vi "Iterate.vi"(8 "error in (no error)":errorcluster, 10 "Iterator Settings":T1={"Prepare timeout (ms)"=200, "Iterate timeout (ms)"=50, "Conclude timeout (ms)"=200, "Iterate period (ms)"=200, "Number of iterations"=5, "Time before stop (ms)"=5, "Active Stop Conditions"={"Number of Iterations"=FALSE, "Time Elapsed"=FALSE, "Iteration Result"=FALSE}, "Prepare Msg"=refnum, "Iterate Msg"=refnum, "Conclude Msg"=refnum, "Iterations End Report"=refnum}, 11 "Iterator Actor in":refnum<class "Iterator NR Actor.lvclass">) -> (0 "error out":errorcluster, 3 "Iterator Actor out":refnum<class "Iterator NR Actor.lvclass">)   [LabVIEW 2023, in "Iterator Actor.lvlib" / "Iterator NR Actor.lvclass"]
doc: "Iteratively calls the Iterate method of the Client. \nStops the iterations either by receiving the Stop signal, or by any of predefined Stop conditions."
uses:
  Iterator NR Actor.lvclass
  Abstract Iterator Actor/Iterator Settings.ctl
  Iterator Actor/Iterator Actor Abstract Messages/Iterator Report Iterations End Msg/Iterator Report Iterations End Msg.lvclass
  <vilib>/ActorFramework/Message/Message.lvclass
  Abstract Iterator Actor/Active Stop Conditions.ctl
  Abstract Iterator Actor/Abstract Iterator Actor.lvclass/Abstract Iterator Actor.ctl
  Abstract Iterator Actor/Stop Reason.ctl
  <vilib>/ActorFramework/Actor/Actor.lvclass/Actor.ctl
  <vilib>/ActorFramework/Message Enqueuer/Message Enqueuer.lvclass/Message Enqueuer.ctl
  Iterator NR Actor.lvclass/Iterator NR Actor.ctl
  <vilib>/ActorFramework/Batch Msg/Batch Msg.lvclass/Batch Msg.ctl
  Abstract Iterator Actor/Iterator Errors.ctl
  Abstract Iterator Actor/Read Stop Iterate Notifier.vi
  <vilib>/ActorFramework/Message Enqueuer/Init from Existing Queue.vi
  <vilib>/ActorFramework/Actor/Read Caller Enqueuer.vi
  <vilib>/ActorFramework/Batch Msg/Send Batch.vi
  <vilib>/ActorFramework/Message Enqueuer/Enqueue.vi
  Iterator NR Actor Messages/Request Iteration Notification Msg/Request Iteration Notification Msg.lvclass
  <vilib>/ActorFramework/Batch Msg/Batch Msg.lvclass
  <userlib>/_OpenG.lib/lvdata/lvdata.llb/LVOOP Is Same Or Descendant Class__ogtk.vi
  <vilib>/ActorFramework/Message Priority Queue/Priority Enqueue.vi
  <vilib>/ActorFramework/Message Enqueuer/Message Enqueuer.lvclass
  Iterator NR Actor Messages/Iteration Msg/Abstract Iteration Msg.lvclass
  <userlib>/_OpenG.lib/time/time.llb/openg_time.lvlib
  Iterator Actor/Iterator Actor Messages/Write Stop Reason Msg/Write Stop Reason Msg.lvclass
  <vilib>/ActorFramework/Actor/Actor.lvclass
  Abstract Iterator Actor/Abstract Iterator Actor.lvclass
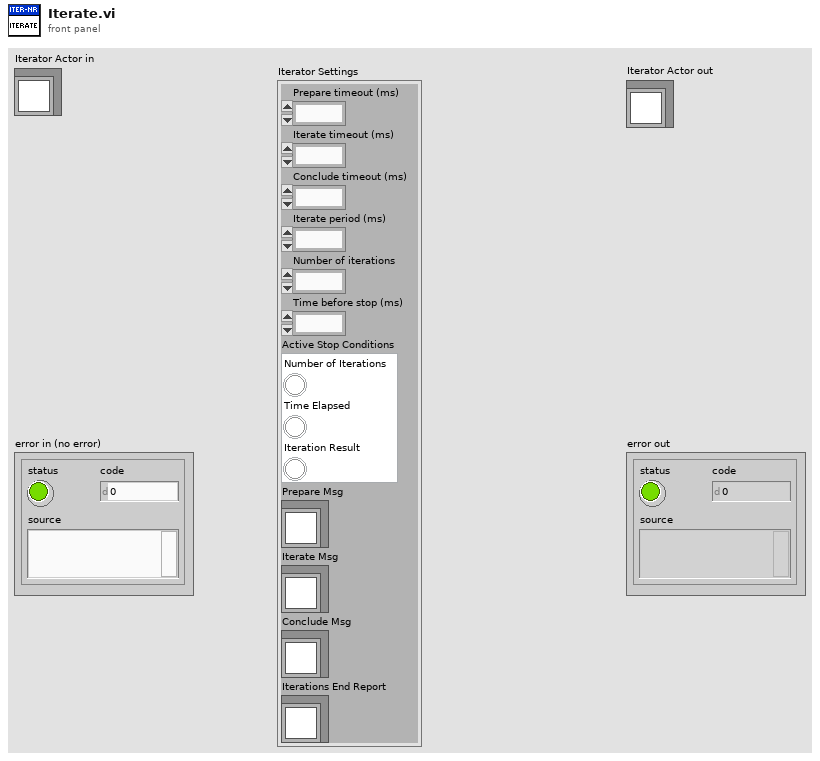
[diagram p1: front panel]
types:
  T1 = typedef "Iterator Actor.lvlib/Abstract Iterator Actor.lvclass/Iterator Settings.ctl" = cluster{"Prepare timeout (ms)":i32, "Iterate timeout (ms)":i32, "Conclude timeout (ms)":i32, "Iterate period (ms)":i32, "Number of iterations":i32, "Time before stop (ms)":i32, "Active Stop Conditions":T2, "Prepare Msg":refnum<class "Message.lvclass">, "Iterate Msg":refnum<class "Message.lvclass">, "Conclude Msg":refnum<class "Message.lvclass">, "Iterations End Report":refnum<class "Iterator Report Iterations End Msg.lvclass">}
  T2 = typedef "Iterator Actor.lvlib/Abstract Iterator Actor.lvclass/Active Stop Conditions.ctl" = cluster{"Number of Iterations":bool, "Time Elapsed":bool, "Iteration Result":bool}
  T3 = typedef "Iterator Actor.lvlib/Abstract Iterator Actor.lvclass/Stop Reason.ctl" = enum16{"Number of Iterations", "Time Elapsed", "Stopped Internally", "Stopped Externally"}
  T4 = typedef "Iterator Actor.lvlib/Abstract Iterator Actor.lvclass/Iterator Errors.ctl" = enum16{"Input parameters are not valid", "Preparation call timed out", "Iteration call timed out", "Conclusion call timed out"}
  T5 = typedef "Iterator Actor.lvlib/Abstract Iterator Actor.lvclass/Stop Condition.ctl" = enum16{"None", "Number of Iterations", "Time Elapsed", "Iteration Result"}
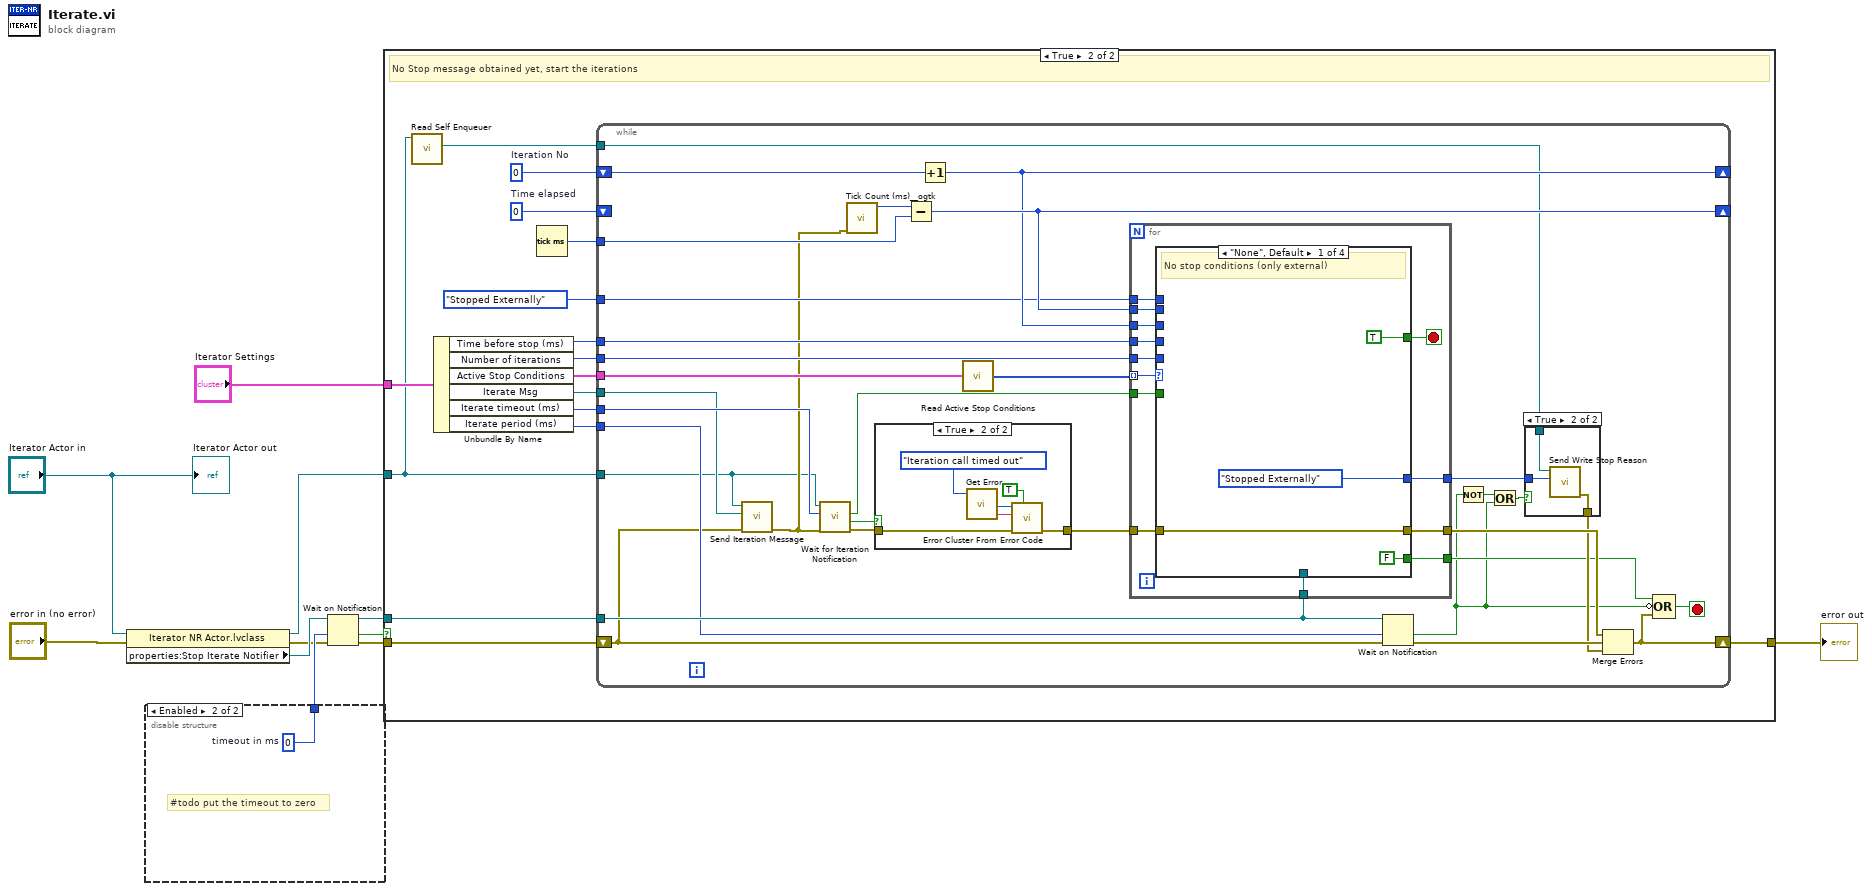
[diagram p0: block diagram]
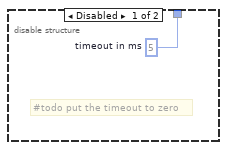
[diagram p2: hidden frame]
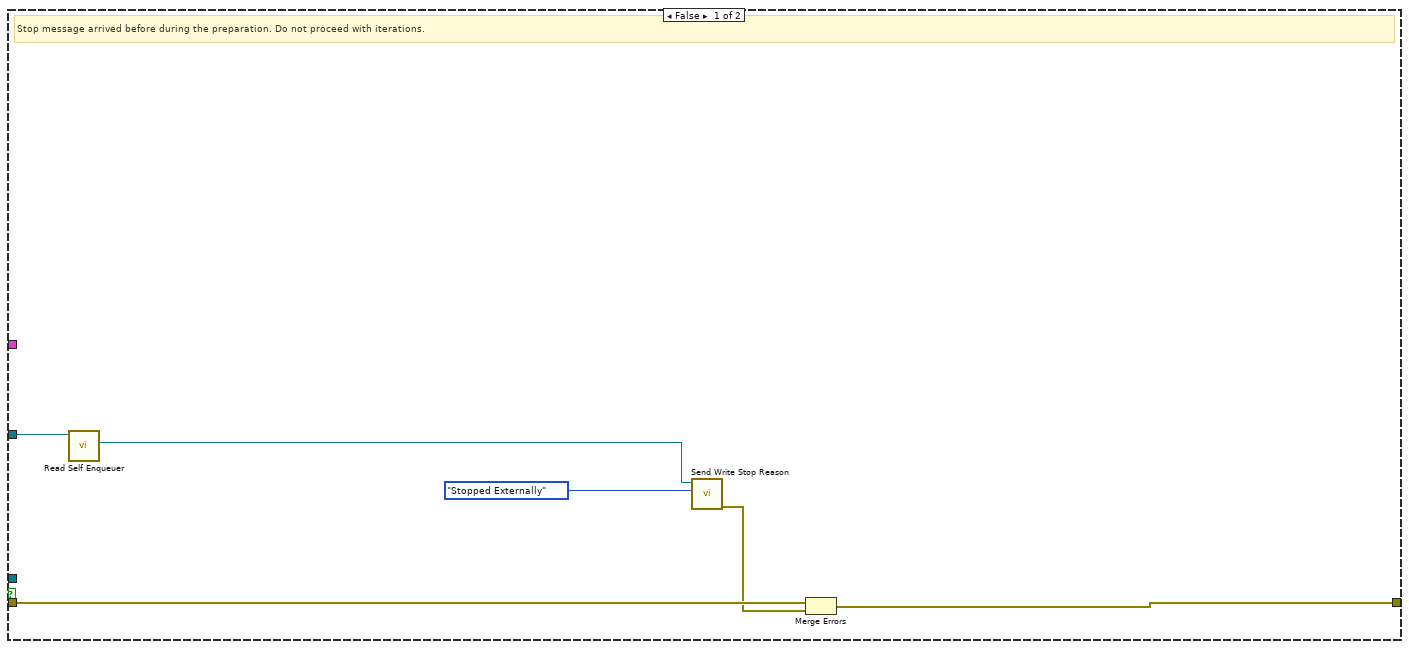
[diagram p3: hidden frame]
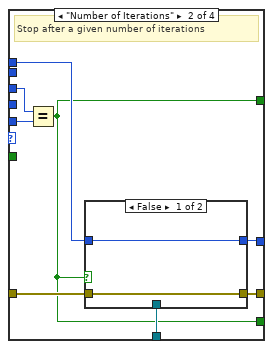
[diagram p4: hidden frame]
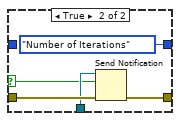
[diagram p5: hidden frame]
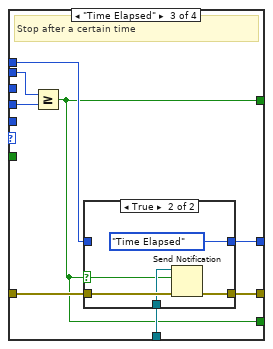
[diagram p6: hidden frame]
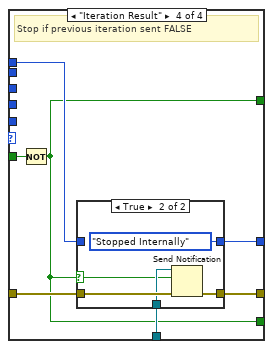
[diagram p8: hidden frame]
diagram:
  n1 = property class="Iterator NR Actor.lvclass"(reference="Iterator Actor in", error in="error in (no error)") -> (reference out=w1:refnum<class "Iterator NR Actor.lvclass">, error out=w3:errorcluster, "properties:Stop Iterate Notifier"=w5:refnum<notifier>)
  n2 = disable-structure shown="Enabled" {
    disable-tunnel: [w12 w13] -> w6
    frame Disabled {
      w12 = 5  # timeout in ms
      # "#todo put the timeout to zero"
    }
    frame Enabled {
      w13 = 0  # timeout in ms
      # "#todo put the timeout to zero"
    }
  }
  n3 = Wait on Notification(notifier=w5, timeout in ms (-1)=w6, error in (no error)=w3) -> (notifier out=w8:refnum<notifier>, timed out?=w7:bool, error out=w9:errorcluster)  [unwired: 1 in, 1 out]
  n4 = case shown="True" w7 {
    tunnel: "Iterator Settings" -> [_ w29]
    tunnel: [w17 w25] -> w10
    tunnel: w9 -> [w19 w24]
    tunnel: w8 -> [_ w23]
    tunnel: w1 -> [w15 w20]
    frame False {
      # "Stop message arrived before during the preparation. Do not proceed with iterations."
      n5 = call <vilib>:"Read Self Enqueuer.vi"("Actor"=w15) -> ("Self Enqueuer"=w14:refnum<class "Message Enqueuer.lvclass">)  [unwired: 10 in]
      n6 = call "Send Write Stop Reason.vi"("Stop Reason"=Stop_Reason."Stopped Externally", "Message Enqueuer in"=w14) -> ("error out"=w16:errorcluster)  [unwired: 8 in, 1 out]
      n7 = Merge Errors(w19, w16) -> (w17:errorcluster)
    }
    frame True {
      w26 = 0  # Iteration No
      w27 = u32 0  # Time elapsed
      # "No Stop message obtained yet, start the iterations"
      n8 = call <vilib>:"Read Self Enqueuer.vi"("Actor"=w20) -> ("Self Enqueuer"=w21:refnum<class "Message Enqueuer.lvclass">)  [unwired: 10 in]
      n9 = Unbundle By Name(w29) -> ("Time before stop (ms)"=w30:i32, "Number of iterations"=w31:i32, "Active Stop Conditions"=w32:T2, "Iterate Msg"=w33:refnum<class "Message.lvclass">, "Iterate timeout (ms)"=w34:i32, "Iterate period (ms)"=w35:i32)
      n10 = Tick Count (ms)() -> (millisecond timer value=w28:u32)
      n11 = while {
        tunnel: w33 -> [w37]
        tunnel: w34 -> [w46]
        tunnel: w35 -> [w54]
        shift-right: [w55] -> w25
        shift-left: w24 -> [w39]
        shift-right: [w57] -> _
        shift-left: w26 -> [w65]
        shift-right: [w58] -> _
        shift-left: w27 -> [_]
        tunnel: w32 -> [w49]
        tunnel: w31 -> [w64]
        tunnel: w30 -> [w63]
        tunnel: w28 -> [w59]
        tunnel: w23 -> [w56]
        tunnel: w21 -> [w53]
        tunnel: Stop_Reason."Stopped Externally" ("Stop Reason") -> [w50]
        tunnel: w20 -> [w36]
        stop <- w62 stop-if-true
        n12 = call "Send Iteration Message.vi"("error in (no error)"=w39, "Iteration Msg"=w37, "Iterator NR Actor in"=w36) -> ("error out"=w38:errorcluster)  [unwired: 8 in]
        n13 = call "Wait for Iteration Notification.vi"("error in (no error)"=w38, "timeout in ms (-1)"=w46, "Iterator NR Actor in"=w36) -> ("error out"=w47:errorcluster, "timed out?"=w44:bool, "Iterate?"=w45:bool)  [unwired: 5 in, 1 out]
        n14 = call <userlib>:"Tick Count (ms)__ogtk.vi"("error in (no error)"=w38) -> ("millisecond timer value"=w60:u32)  [unwired: 9 in, 1 out]
        n15 = case shown="True" w44 {
          tunnel: w47 -> [w132 w135]
          tunnel: [w132 w134] -> w61
          frame False {
          }
          frame True {
            n16 = call "Get Error.vi"("Error"=Iterator_Errors."Iteration call timed out") -> ("source"=w137:string, "code"=w136:i32)  [unwired: 2 in, 1 out]
            n17 = call <vilib>:"Error Cluster From Error Code.vi"("show call chain? (False)"=TRUE ("is warning? (False)"), "error in (no error)"=w135, "error message (\"\")"=w137, "error code (0)"=w136) -> ("error out"=w134:errorcluster)  [unwired: 5 in]
          }
        }
        n18 = Subtract(x=w60, y=w59) -> (x-y=w58:u32)
        n19 = Increment(x=w65) -> (x+1=w57:i32)
        n20 = call "Read Active Stop Conditions.vi"("Active Stop Conditions"=w49) -> ("Active Stop Conditions"=w48:T5[])
        n21 = for {
          tunnel: w48 -> [w79] mode=indexing
          tunnel: w64 -> [w78]
          tunnel: w63 -> [w77]
          tunnel: w58 -> [w75]
          tunnel: w57 -> [w74]
          tunnel: w45 -> [w73]
          tunnel: w56 -> [w72]
          tunnel: w61 -> [w76]
          tunnel: [w80] -> w66
          tunnel: w50 -> [w70]
          tunnel: [w71] -> w52
          tunnel: [w68] -> w43
          stop <- w69 stop-if-true
          n22 = case shown="\"None\", Default" w79 {
            tunnel: w76 -> [w84 w90 w107 w119]
            tunnel: [w84 w89 w106 w121] -> w80
            tunnel: w72 -> [_ w92 w105 w120]
            tunnel: w78 -> [_ w91 _ _]
            tunnel: w77 -> [_ _ w104 _]
            tunnel: w75 -> [_ _ w103 _]
            tunnel: w74 -> [_ w88 _ _]
            tunnel: w73 -> [_ _ _ w116]
            tunnel: [Stop_Reason."Stopped Externally" ("Stop Reason") w87 w102 w118] -> w71
            tunnel: w70 -> [_ w86 w101 w117]
            tunnel: [TRUE ("Reply") w85 w100 w115] -> w69
            tunnel: [FALSE w85 w100 w115] -> w68
            frame "None", Default {
              # "No stop conditions (only external)"
            }
            frame "Number of Iterations" {
              # "Stop after a given number of iterations"
              n23 = Equal?(x=w88, y=w91) -> (x = y?=w85:bool)
              n24 = case shown="False" w85 {
                selector: w85 -> [_ w96]
                tunnel: w92 -> [_ w97]
                tunnel: w90 -> [w94 w99]
                tunnel: [w94 w98] -> w89
                tunnel: [w93 Stop_Reason."Number of Iterations" ("Stop Reason")] -> w87
                tunnel: w86 -> [w93 _]
                frame False {
                }
                frame True {
                  n25 = Send Notification(notification=w96, notifier=w97, error in (no error)=w99) -> (error out=w98:errorcluster)  [unwired: 1 out]
                }
              }
            }
            frame "Time Elapsed" {
              # "Stop after a certain time"
              n26 = Greater Or Equal?(x=w103, y=w104) -> (x >= y?=w100:bool)
              n27 = case shown="True" w100 {
                selector: w100 -> [_ w111]
                tunnel: w105 -> [_ w112]
                tunnel: w107 -> [w109 w114]
                tunnel: [w109 w113] -> w106
                tunnel: [w108 Stop_Reason."Time Elapsed" ("Stop Reason")] -> w102
                tunnel: w101 -> [w108 _]
                frame False {
                }
                frame True {
                  n28 = Send Notification(notification=w111, notifier=w112, error in (no error)=w114) -> (error out=w113:errorcluster)  [unwired: 1 out]
                }
              }
            }
            frame "Iteration Result" {
              # "Stop if previous iteration sent FALSE"
              n29 = Not(x=w116) -> (.not. x?=w115:bool)
              n30 = case shown="True" w115 {
                selector: w115 -> [_ w125]
                tunnel: w120 -> [_ w126]
                tunnel: w119 -> [w123 w128]
                tunnel: [w123 w127] -> w121
                tunnel: [w122 Stop_Reason."Stopped Internally" ("Stop Reason")] -> w118
                tunnel: w117 -> [w122 _]
                frame False {
                }
                frame True {
                  n31 = Send Notification(notification=w125, notifier=w126, error in (no error)=w128) -> (error out=w127:errorcluster)  [unwired: 1 out]
                }
              }
            }
          }
        }
        n32 = Wait on Notification(notifier=w56, timeout in ms (-1)=w54, error in (no error)=w39) -> (timed out?=w41:bool, error out=w67:errorcluster)  [unwired: 1 in, 2 out]
        n33 = Not(x=w41) -> (.not. x?=w40:bool)
        n34 = Or(x=w40, y=w41) -> (x .or. y?=w42:bool)
        n35 = case shown="True" w42 {
          tunnel: w53 -> [_ w131]
          tunnel: w52 -> [_ w130]
          tunnel: [_ w129] -> w51
          frame False {
          }
          frame True {
            n36 = call "Send Write Stop Reason.vi"("Stop Reason"=w130, "Message Enqueuer in"=w131) -> ("error out"=w129:errorcluster)  [unwired: 8 in, 1 out]
          }
        }
        n37 = Merge Errors(w66, w67, w51) -> (w55:errorcluster)
        n38 = Compound Arithmetic op=OR(w43, invert w41, w55) -> (w62:bool)
      }
    }
  }
  "error out" <- w10
  "Iterator Actor out" <- "Iterator Actor in"
